vi "AcquireImage.vi"(5 "Image Name":string="untitled", 7 "error in":errorcluster, 8 "Contrast":dbl, 9 "Brightness":i64, 10 "Session In":T1) -> (0 "error out":errorcluster, 2 "Image":T2(plugin-control), 3 "Session Out":T1)   [LabVIEW 2017]
uses:
  <vilib>/userdefined/High Color/IMAQdx.ctl
  <vilib>/vision/driver/NI_Vision_Acquisition_Software.lvlib
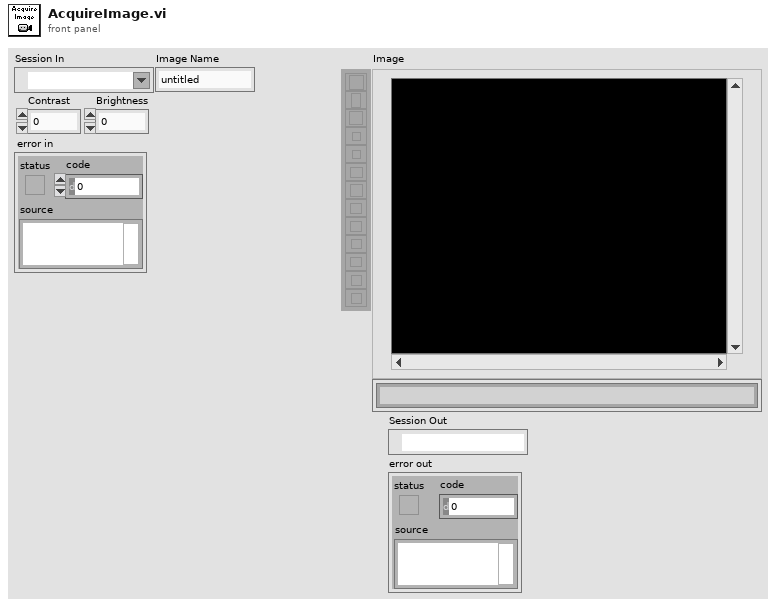
[diagram p1: front panel]
types:
  T1 = typedef "IMAQdx.ctl" = refnum<k21>
  T2 = typedef "IMAQ Image.ctl" = refnum<image>
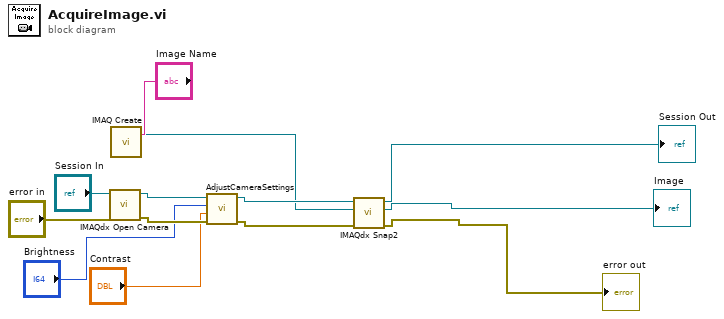
[diagram p0: block diagram]
diagram:
  n1 = call <vilib>:"IMAQdx Open Camera.vi"("error in"="error in", "Session In"="Session In") -> ("error out"=w8:errorcluster, "Session Out"=w11:T1)  [unwired: 8 in]
  n2 = call "IMAQ Create"("Image Name"="Image Name") -> ("New Image"=w9:T2)  [unwired: 4 in, 1 out]
  n3 = call "AdjustCameraSettings.vi"("error in (no error)"=w8, "Contrast"="Contrast", "Brightness"="Brightness", "Session In"=w11) -> ("error out"=w7:errorcluster, "IMAQdx Session"=w10:T1)  [unwired: 4 in, 2 out]
  n4 = call <vilib>:"IMAQdx Snap2.vi"("error in"=w7, "Image In"=w9, "Session In"=w10) -> ("error out"=→"error out":errorcluster, "Image Out"=→"Image":T2, "Session Out"=→"Session Out":T1)  [unwired: 6 in]
